vi "LungBriteFront.vi"() -> ()   [LabVIEW 2019]
doc: "Use this template to build a simple state machine design pattern. Each state executes code and determines which state to transition to."
uses:
  controls/State.ctl
  controls/Data.ctl
  <vilib>/myRIO/Instrument Drivers/Onboard IO/AI/AI.lvlib
  <vilib>/myRIO/Instrument Drivers/Utilities/Utilities.lvlib
  <vilib>/myRIO/Express VI/Onboard Devices/Button/Button Express VI.xnode
  <vilib>/myRIO/Instrument Drivers/Onboard IO/DIO/vis/Read.vi
  <vilib>/myRIO/Instrument Drivers/Onboard IO/DIO/DIO.lvlib
  <vilib>/myRIO/Common/Instrument Driver Framework/myRIO v1.0/DIO/typedefs/DIO Channels Enum.ctl
  <vilib>/myRIO/Common/Instrument Driver Framework/myRIO v1.0/DIO/typedefs/DIO Channels List.ctl
  <vilib>/myRIO/Common/Instrument Driver Framework/Utilities/typedefs/Generic FPGA Reference.ctl
  <vilib>/myRIO/Common/Instrument Driver Framework/Utilities/typedefs/myRIO v1.0 Reference.ctl
  <vilib>/myRIO/Common/Instrument Driver Framework/Utilities/typedefs/Hardware Version Enum.ctl
  <vilib>/myRIO/Common/Instrument Driver Framework/Utilities/typedefs/myRIO Generic Hardware Reference.ctl
  <vilib>/myRIO/Instrument Drivers/Onboard IO/DIO/typedefs/DIO Reference.ctl
  <vilib>/myRIO/Instrument Drivers/Onboard IO/DIO/vis/myRIO DIO Open.xnode
  <vilib>/myRIO/Common/Instrument Driver Framework/Utilities/vis/Is FPGA Ref Available.vi
  <vilib>/myRIO/Common/Instrument Driver Framework/myRIO v1.0/DIO/vis/myRIO v1.1 Open DIO.vi
  <vilib>/userDefined/High Color/nirio_resource_hc.ctl
panel:
  out "Next State":T1
  in  "Channel Names 2":tag[](array[tag])=["C/AI1"]
  in  "Exit":bool
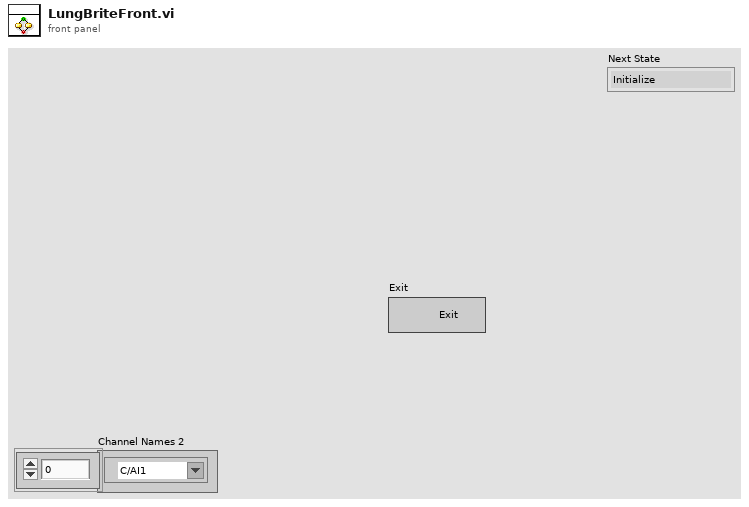
[diagram p1: front panel]
types:
  T1 = typedef "State.ctl" = enum16{"Initialize", "Wait for Event", "Read Sound", "Report", "No Breathing Detected", "Emergency Contact", "Exit"}
  T2 = typedef "Data.ctl" = cluster{"STOP":bool, "Seconds of No Breathing":dbl, "No Breathing":dbl}
  T3 = typedef "AI.lvlib/AI Reference.ctl" = cluster{"myRIO Reference":T4, "AI Channels List":T8, "AI Scaling Constants List":T10}
  T4 = typedef "myRIO Generic Hardware Reference.ctl" = cluster{"myRIO Model":T5, "myRIO Hardware Reference":T6}
  T5 = typedef "Hardware Version Enum.ctl" = enum16{"Unknown", "myRIO-1900", "myRIO-1950", "roboRIO", "NI ELVIS RIO CM", "ELVIS III"}
  T6 = typedef "myRIO v1.0 Reference.ctl" = cluster{"Generic FPGA Reference":T7, "Allow multiple opens":bool}
  T7 = typedef "Generic FPGA Reference.ctl" = refnum<k20>
  T8 = typedef "AI Channels List.ctl" = T9[]
  T9 = typedef "AI Channels Enum.ctl" = enum16{"Not Connected", "AudioIn/Left", "AudioIn/Right", "C/AI0", "C/AI1", "A/AI0", "A/AI1", "A/AI2", "A/AI3", "A/AI4", "A/AI5", "A/AI6", "A/AI7", "B/AI0", "B/AI1", "B/AI2", "B/AI3", "B/AI4", "B/AI5", "B/AI6", "B/AI7", "AI/AI0", "AI/AI1", "AI/AI2", "AI/AI3", "A/AI0 (DIFF)", "A/AI1 (DIFF)", "A/AI2 (DIFF)", "A/AI3 (DIFF)", "B/AI0 (DIFF)", "B/AI1 (DIFF)", "B/AI2 (DIFF)", "B/AI3 (DIFF)"}
  T10 = typedef "Analog Scaling Constants List.ctl" = T11[]
  T11 = typedef "Analog Scaling Constants.ctl" = cluster{"LSB Weight (Volts)":dbl, "Offset (Volts)":dbl, "Signed?":bool}
  T12 = enum16{"open", "replace", "create", "open or create", "replace or create", "replace or create with confirmation"}
  T13 = typedef "DIO.lvlib/DIO Reference.ctl" = cluster{"myRIO Reference":T4, "DIO Channels List":T14}
  T14 = typedef "DIO Channels List.ctl" = T15[]
  T15 = typedef "DIO Channels Enum.ctl" = enum16{"Not Connected", "C/DIO0", "C/DIO1", "C/DIO2", "C/DIO3", "C/DIO4", "C/DIO5", "C/DIO6", "C/DIO7", "A/DIO0", "A/DIO1", "A/DIO2", "A/DIO3", "A/DIO4", "A/DIO5", "A/DIO6", "A/DIO7", "A/DIO8", "A/DIO9", "A/DIO10", "A/DIO11", "A/DIO12", "A/DIO13", "A/DIO14", "A/DIO15", "A/DIO16", "A/DIO17", "A/DIO18", "A/DIO19", "B/DIO0", "B/DIO1", "B/DIO2", "B/DIO3", "B/DIO4", "B/DIO5", "B/DIO6", "B/DIO7", "B/DIO8", "B/DIO9", "B/DIO10", "B/DIO11", "B/DIO12", "B/DIO13", "B/DIO14", "B/DIO15", "B/DIO16", "B/DIO17", "B/DIO18", "B/DIO19", "LED0", "LED1", "LED2", "LED3", "Button0", "DIO/DIO0", "DIO/DIO1", "DIO/DIO2", "DIO/DIO3", "DIO/DIO4", "DIO/DIO5", "DIO/DIO6", "DIO/DIO7", "DIO/DIO8", "DIO/DIO9", "SPI/CS0", "SPI/CS1", "SPI/CS2", "SPI/CS3", "LED RADIO (Green)", "LED RADIO (Red)", "LED COMM (Green)", "LED COMM (Red)", "LED MODE (Green)", "LED MODE (Red)"}
  T16 = typedef "nirio_resource_hc.ctl" = tag
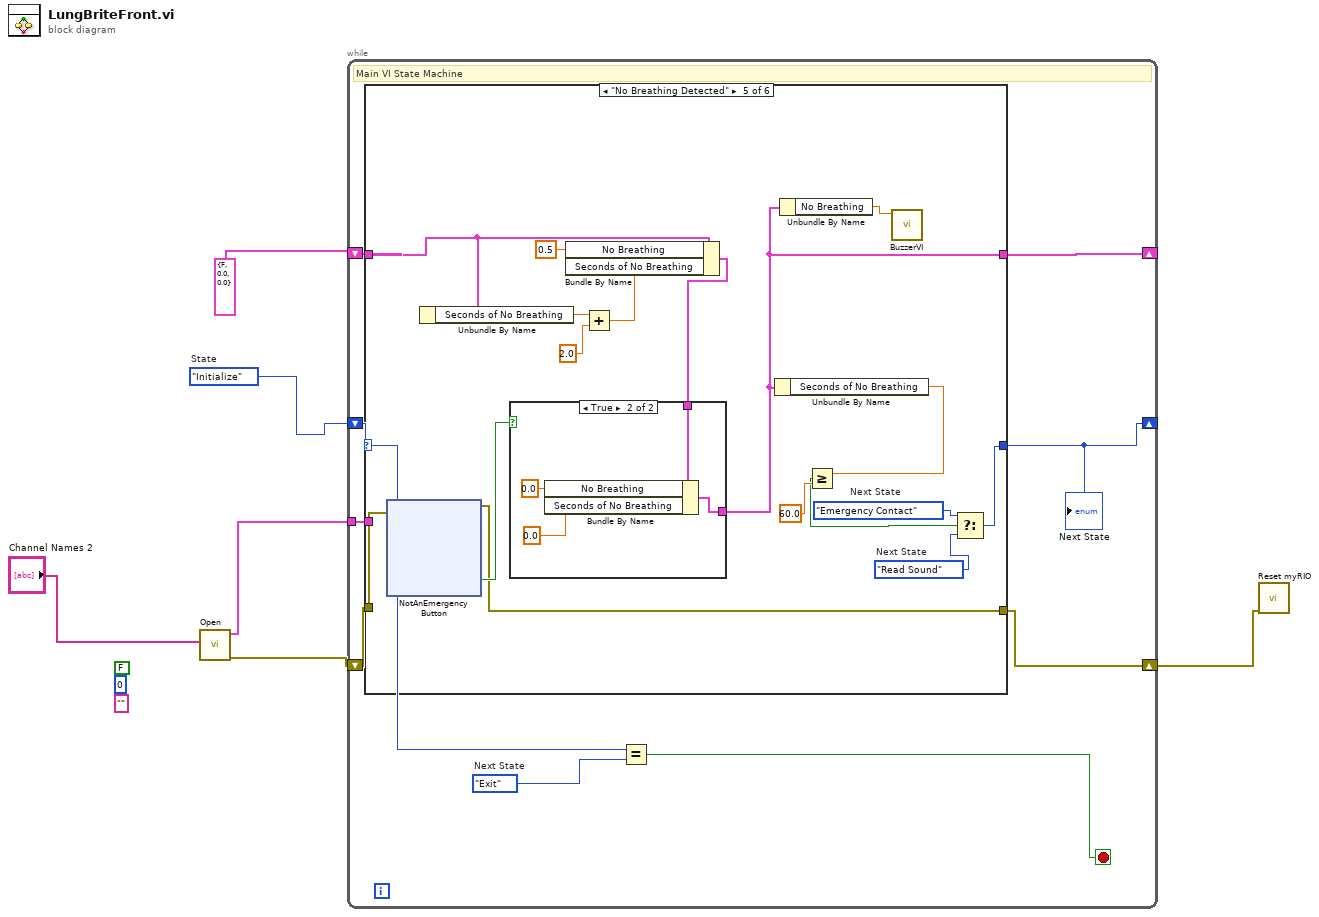
[diagram p0: block diagram]
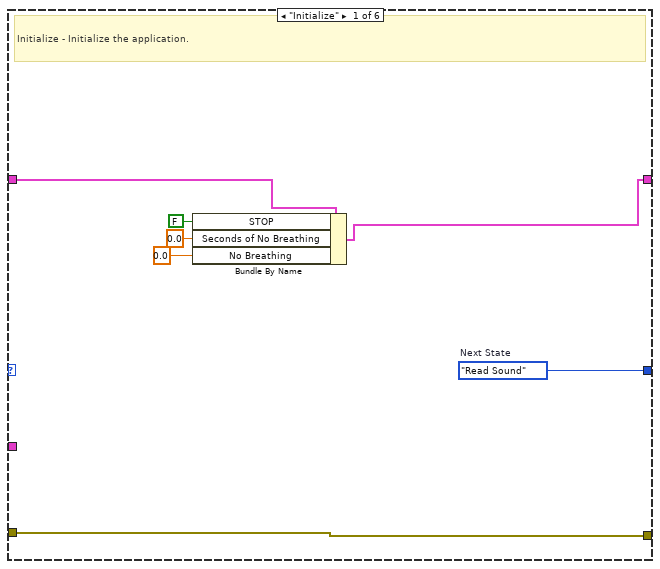
[diagram p2: hidden frame]
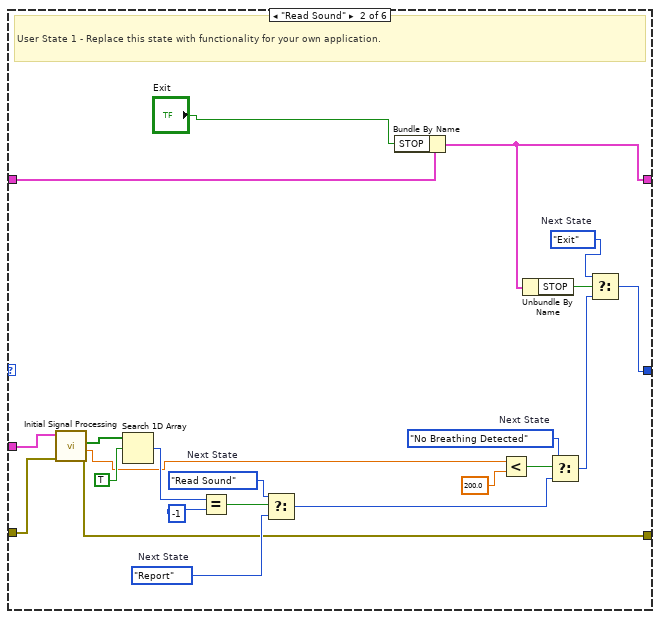
[diagram p3: hidden frame]
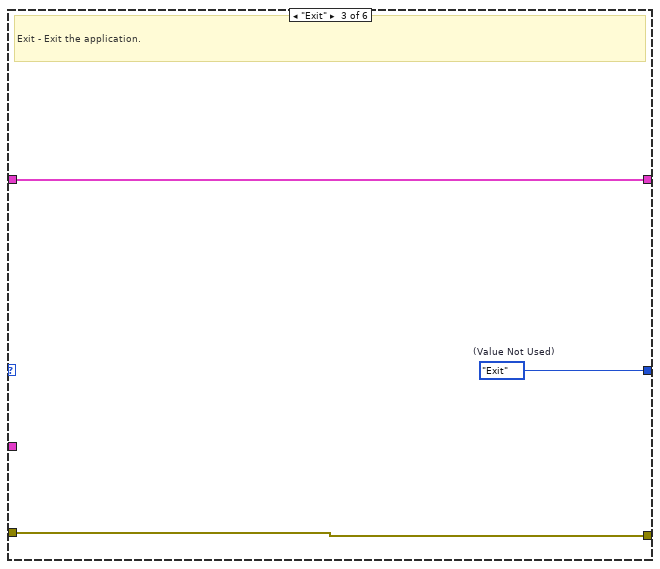
[diagram p4: hidden frame]
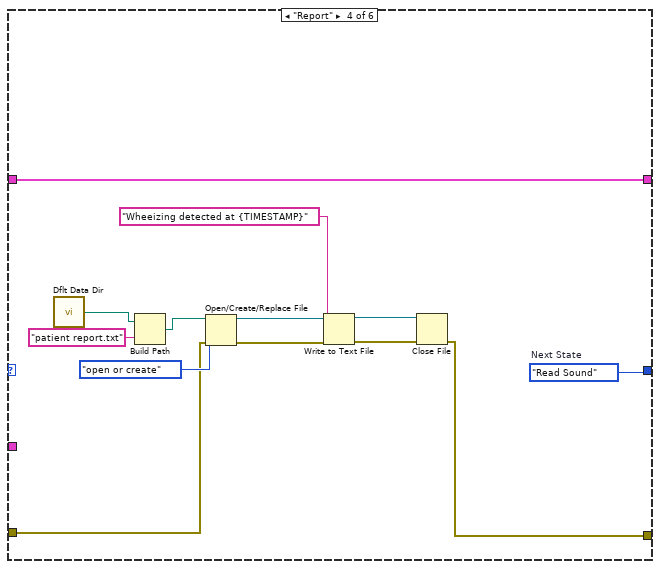
[diagram p5: hidden frame]
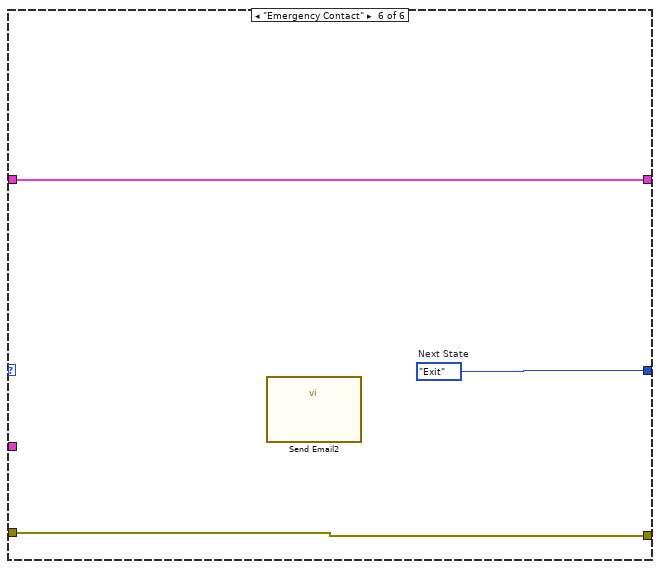
[diagram p7: hidden frame]
diagram:
  (unwired) FALSE ("status")
  (unwired) 0 ("code")
  (unwired) "" ("source")
  w5 = State."Initialize"  # State
  n1 = call <vilib>:"Open.vi"("Channel Names"="Channel Names 2") -> ("error out"=w2:errorcluster, "AI Ref Out"=w1:T3)  [unwired: 9 in]
  n2 = while {
    shift-right: [w14] -> _
    shift-left: T2 {"STOP"=FALSE, "Seconds of No Breathing"=0.0, "No Breathing"=0.0} ("Data") -> [w15]
    shift-right: [w11] -> _
    shift-left: w5 -> [w12]
    tunnel: w1 -> [w8]
    shift-right: [w9] -> w3
    shift-left: w2 -> [w7]
    stop <- w10 stop-if-true
    w13 = State."Exit"  # Next State
    # "Main VI State Machine"
    n3 = case shown="\"No Breathing Detected\"" w12 {
      tunnel: w15 -> [w20 w31 w47 w50 w77 w120]
      tunnel: [w16 w30 w47 w50 w65 w120] -> w14
      tunnel: [w22 w42 w46 w51 w68 w119] -> w11
      tunnel: [w21 w25 w45 w49 w61 w118] -> w9
      tunnel: w8 -> [_ w26 _ _ _ _]
      tunnel: w7 -> [w21 w24 w45 w48 w62 w118]
      frame "Initialize" {
        w22 = State."Read Sound"  # Next State
        # "Initialize - Initialize the application."
        n4 = Bundle By Name(cluster=w20, "STOP"=FALSE, "Seconds of No Breathing"=0.0, "No Breathing"=0.0) -> (w16:T2)
      }
      frame "Read Sound" {
        w33 = State."Read Sound"  # Next State
        w38 = State."No Breathing Detected"  # Next State
        w34 = State."Report"  # Next State
        w43 = State."Exit"  # Next State
        # "User State 1 - Replace this state with functionality for your own application."
        n5 = call "Initial Signal Processing.vi"("error in"=w24, "AI Ref In"=w26) -> ("error out"=w25:errorcluster, "max value"=w27:dbl, "Wheeze?"=w29:bool[])  [unwired: 6 in, 1 out]
        n6 = Search 1D Array(1D array=w29, element=TRUE) -> (index of element=w37:i32)  [unwired: 1 in]
        n7 = Equal?(x=w37, y=-1) -> (x = y?=w35:bool)
        n8 = Select(t=w33, s=w35, f=w34) -> (s? t:f=w32:T1)
        n9 = Bundle By Name(cluster=w31, "STOP"="Exit") -> (w30:T2)
        n10 = Less?(x=w27, y=200.0) -> (x < y?=w40:bool)
        n11 = Unbundle By Name(w30) -> ("STOP"=w44:bool)
        n12 = Select(t=w38, s=w40, f=w32) -> (s? t:f=w39:T1)
        n13 = Select(t=w43, s=w44, f=w39) -> (s? t:f=w42:T1)
      }
      frame "Exit" {
        w46 = State."Exit"  # (Value Not Used)
        # "Exit - Exit the application."
      }
      frame "Report" {
        w51 = State."Read Sound"  # Next State
        n14 = call <vilib>:"Dflt Data Dir.vi"() -> ("App:Default Data Directory"=w60:path)
        n15 = Build Path(base path=w60, name or relative path="patient report.txt") -> (appended path=w58:path)
        n16 = Open/Create/Replace File(file path (use dialog)=w58, error in=w48, operation (0:open)=T12."open or create") -> (refnum out=w56:refnum<file>, error out=w53:errorcluster)  [unwired: 3 in, 1 out]
        n17 = Write to Text File(file (use dialog)=w56, text="Wheeizing detected at {TIMESTAMP}", error in=w53) -> (refnum out=w54:refnum<file>, error out=w52:errorcluster)  [unwired: 1 in, 1 out]
        n18 = Close File(refnum=w54, error in=w52) -> (error out=w49:errorcluster)  [unwired: 1 out]
      }
      frame "No Breathing Detected" {
        w69 = State."Emergency Contact"  # Next State
        w70 = State."Read Sound"  # Next State
        n19 = xnode "NotAnEmergencyButton"("error in (no error)"=w62) -> ("Value"=w63:bool, "error out"=w61:errorcluster)
        n20 = Unbundle By Name(w77) -> ("Seconds of No Breathing"=w76:dbl)
        n21 = Add(x=w76, y=2.0) -> (x+y=w75:dbl)
        n22 = Bundle By Name(cluster=w77, "No Breathing"=0.5, "Seconds of No Breathing"=w75) -> (w66:T2)
        n23 = case shown="True" w63 {
          tunnel: w66 -> [w113 w117]
          tunnel: [w113 w116] -> w65
          frame False {
          }
          frame True {
            n24 = Bundle By Name(cluster=w117, "No Breathing"=0.0, "Seconds of No Breathing"=0.0) -> (w116:T2)
          }
        }
        n25 = Unbundle By Name(w65) -> ("Seconds of No Breathing"=w73:dbl)
        n26 = Unbundle By Name(w65) -> ("No Breathing"=w67:dbl)
        n27 = Greater Or Equal?(x=w73, y=60.0) -> (x >= y?=w71:bool)
        n28 = call "BuzzerVI.vi"("Duty Cycle"=w67) -> ()  [unwired: 11 in]
        n29 = Select(t=w69, s=w71, f=w70) -> (s? t:f=w68:T1)
      }
      frame "Emergency Contact" {
        w119 = State."Exit"  # Next State
        n30 = call "Send Email2"() -> ()  [unwired: 11 in, 1 out]
      }
    }
    "Next State" <- w11
    n31 = Equal?(x=w12, y=w13) -> (x = y?=w10:bool)
  }
  n32 = call <vilib>:"Reset myRIO.vi"("error in (no error)"=w3) -> ()  [unwired: 10 in, 1 out]
